vi "PID control - Circle cjehf.vi"() -> ()   [LabVIEW 2017]
uses:
  <vilib>/Simulation/Scripting/Companion Diagram/SimConfigNode/SimParams.ctl
  <vilib>/Simulation/Scripting/Companion Diagram/SimConfigNode/_simSolvers.ctl
  <vilib>/Simulation/Implementation/Shared/SIMSCR Execution Mode.ctl
  <vilib>/Simulation/Param Hierarchy/Typedefs/SIMPH Param Control Actions.ctl
  <vilib>/Simulation/Implementation/Shared/NILVSim_ParamChanged.vi
  <vilib>/Simulation/Implementation/Shared/NILVSIM_BeginStep.vi
  <vilib>/Simulation/Implementation/Shared/NILVSim_Manager.vi
  <vilib>/Utility/error.llb/Clear Errors.vi
  <vilib>/Simulation/Implementation/Shared/NILVSim_FinalizeModel.vi
  <vilib>/DAQmx/read.llb/DAQmx Read (Counter DBL 1Chan 1Samp).vi
  <vilib>/DAQmx/read.llb/DAQmx Read (Digital Bool 1Line 1Point).vi
  917b7e52-755f-4d44-bea8-9e7c9beac24e.vi
  a58f9967-76f1-4ebc-ad3d-26e75a3ca160.vi
  <vilib>/DAQmx/write.llb/DAQmx Write (Analog DBL 1Chan 1Samp).vi
  <vilib>/DAQmx/create/channels.llb/DAQmx Create Channel (AO-Voltage-Basic).vi
  <vilib>/DAQmx/create/channels.llb/DAQmx Create Channel (DI-Digital Input).vi
  <vilib>/DAQmx/create/channels.llb/DAQmx Create Channel (CI-Count Edges).vi
  <vilib>/Simulation/Implementation/Shared/SIM Unbundle Sim Info.vi
  <vilib>/Simulation/Implementation/Shared/NILVSim_Initialize.vi
  <vilib>/Simulation/Utility/Implementation/NILVSim Get Time and IsAcceptedStep.vi
  <vilib>/Simulation/Implementation/Shared/SIMSH Read Queue.vi
  <vilib>/Simulation/Implementation/Shared/NILVSim_GetModelError.vi
  <vilib>/Simulation/Implementation/Shared/SIM Bundle Sim Info.vi
  <vilib>/DAQmx/miscellaneous.llb/DAQmx Fill In Error Info.vi
  <vilib>/Simulation/Implementation/XNodeFramework/SimXNode/SimX.xnode
  <vilib>/Simulation/Model Libraries/PID/SIM PID (Parallel).vi
  <vilib>/Simulation/Model Libraries/PID/SIM PID.vi
  <vilib>/Simulation/Scripting/Companion Diagram/SimConfigNode/SimDog.xnode
  <vilib>/Simulation/Model Libraries/PID/SIM PID (Academic).vi
  <vilib>/Simulation/Implementation/Shared/NI_SIM_Implementation.lvlib
panel:
  out "index":dbl
  out "x check":dbl
  out "stop":bool
  out "y final check":dbl
  out "y check":dbl
  out "array x Length":dbl
  out "X array":dbl[](array[numeric])
  out "array Y length":dbl
  out "Y array":dbl[](array[numeric])
  out "Numeric y":dbl
  out "Numeric x":dbl
  out "Numeric 2":dbl
  in  "Radius":dbl
  out "led check":bool
  in  "check instruc":bool
  out "down 2":bool
  out "down":bool
  out "right":bool
  out "x entered":dbl
  out "y enetred":dbl
  out "greater -1 x":bool
  out "less 1 x":bool
  out "direction selected":dbl
  out "circle reset":bool
  in  "part circle":T1(ring)=enum."a"
  out "at 2f":bool
  out "Step 2J":bool
  out "Step 2H":bool
  out "Shape drawing steps":enum16{"corner", "1st switch", "reverse"}(ring)
  out "Step 2D":bool
  out "Step 2C":bool
  out "c":bool
  in  "height":dbl
  in  "length":dbl
  in  "part":T2(ring)=enum."a"
  out "Step 2A":bool
  out "Step 2B":bool
  in  "Has encoders been reset?":enum16{"don't reset", "reset"}(ring)
  out "x distance currently being travelled":dbl
  out "y distance currently being travelled":dbl
  out "error calced":dbl
  out "p1 dis 2":dbl
  out "p1 dis":dbl
  out "error y":dbl
  out "calc distance y":dbl
  out "calc distanc x":dbl
  out "error x":dbl
  out "reached y":bool
  out "reached x":bool
  out "Numeric":dbl
  in  "Draw rectangle":bool
  in  "Draw circle":bool
  out "In drawing mode":bool
  in  "Right-Down":bool
  in  "Left-Up":bool
  in  "Left-Down":bool
  in  "Right-Up":bool
  in  "right":bool
  in  "left":bool
  in  "motor 2":dbl(slide)=1.5 scale=-10.0..10.0
  in  "down":bool
  in  "up":bool
  in  "Y Length":dbl=30.0
  in  "X Length":dbl=30.0
  in  "Motor 2 encoder":tag="Dev1/ctr1"
  out "Pulses M2":dbl format="%.2f"
  in  "Motor 1 encoder":tag="Dev1/ctr0"
  out "Pulses M1":dbl format="%.2f"
  out "Right":bool
  out "Bottom":bool
  out "Left":bool
  out "Top":bool
  in  "Switch 4/Line 3":tag="Dev1/port0/line3"
  in  "Switch 3/Line 2":tag="Dev1/port0/line2"
  in  "Switch 2/Line 1":tag="Dev1/port0/line1"
  in  "Switch 1/Line 0":tag="Dev1/port0/line0"
  in  "Motor stop":bool
  in  "Motor 1":tag="Dev1/ao0"
  in  "max Voltage":dbl=10.0
  in  "Min Voltage":dbl=-10.0
  in  "Motor 2":tag="Dev1/ao1"
  in  "motor 1":dbl(slide)=1.5 scale=-10.0..10.0
  in  "stop":bool
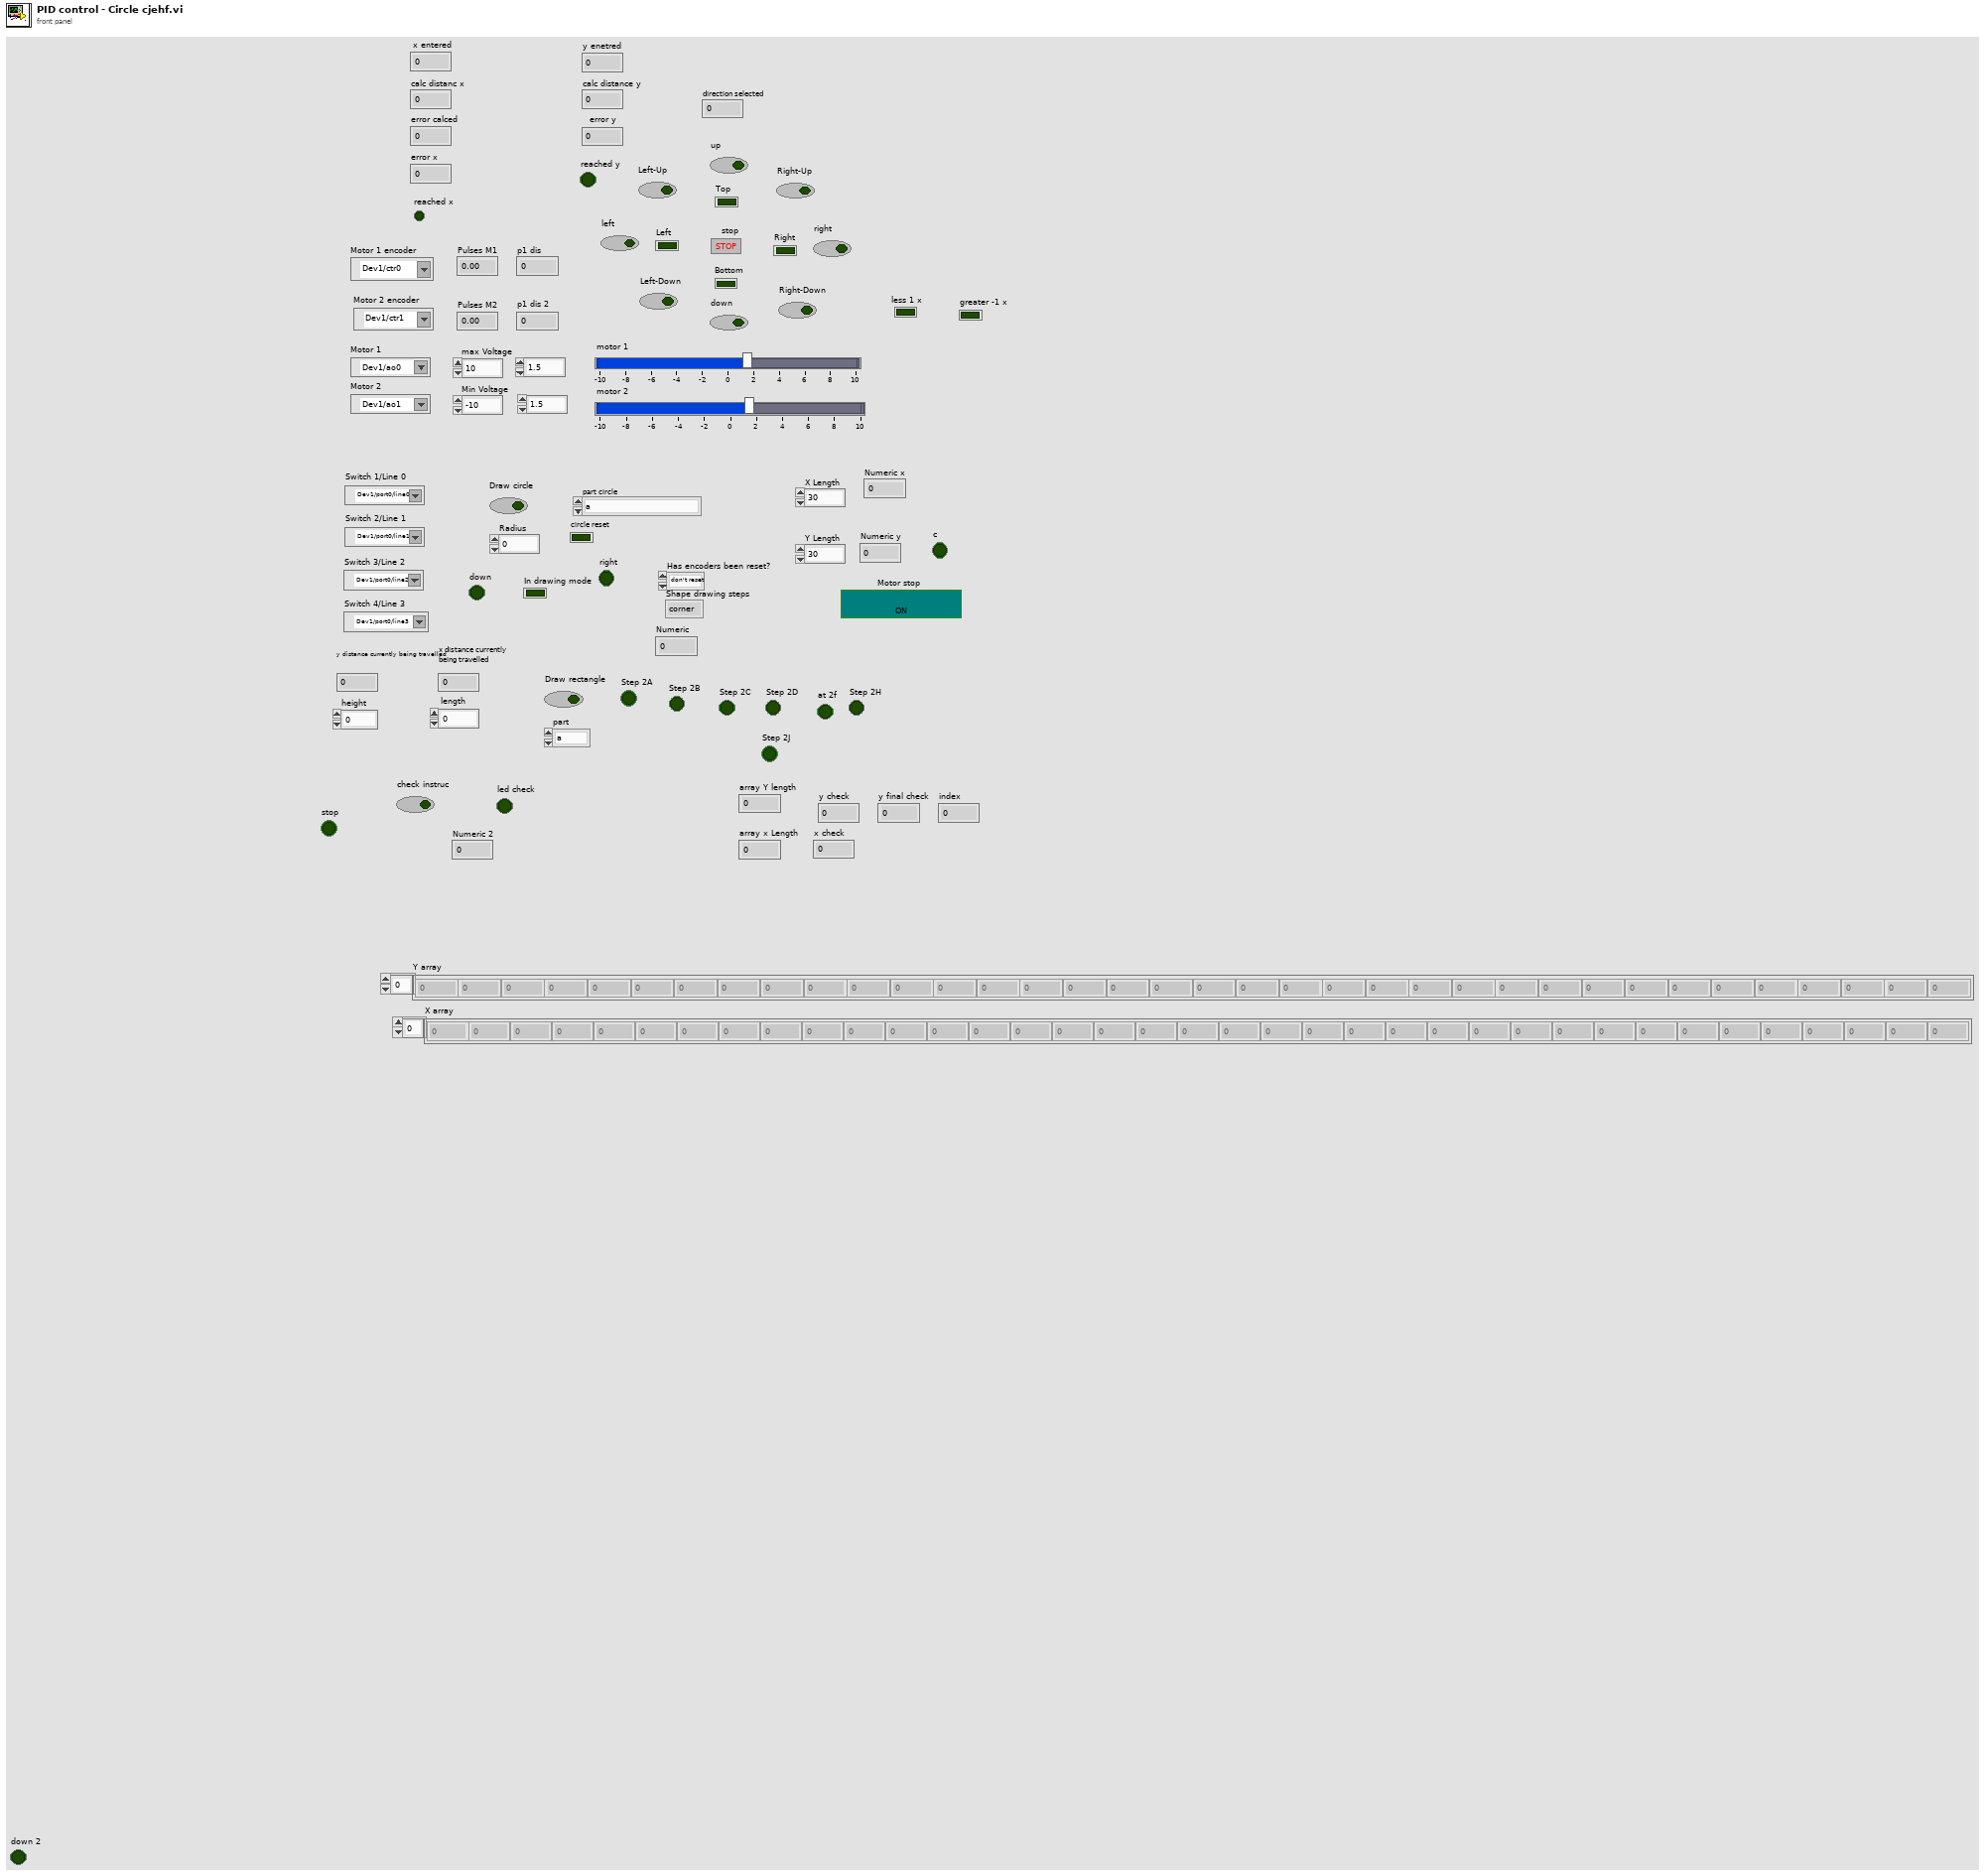
[diagram p1: front panel]
types:
  T1 = enum16{"nothing", "circle", "reset_before_circle", "radius_travel", "going right", "going down", "a"}
  T2 = enum16{"nothing", "j", "i", "h", "g", "f", "e", "d", "c", "b", "a"}
  T3 = enum16{"Simulate to Completion", "Single Time-Step Simulation (Fixed Step Only)"}
  T4 = typedef "SIMSCR Execution Mode.ctl" = enum16{"Simulate to Completion", "Single Time-Step Simulation (Fixed Step Only)"}
  T5 = typedef "SIMPH Param Control Actions.ctl" = enum16{"get params", "set params"}
  T6 = cluster{"SIMSH Sim Time":dbl, "SIM PID Derivative Gain.vi":cluster{"output":dbl}, "SIM PID Derivative Gain.vi - SIMSH":cluster{"SIMSH Sim Time":dbl, "t 3":dbl, "Select 2":cluster{"s? t:f":dbl}, "Equal?":cluster{"x = y?":bool}, "Or":cluster{"x .or. y?":bool}, "Equal To 0?":cluster{"x = 0?":bool}}, "High Frequency [s] (Tf)":dbl, "Gain":cluster{"output":dbl}, "Summation":cluster{"Result":dbl}, "Integral Gain - series.vi":cluster{"output":dbl}, "Integral Gain - series.vi - SIMSH":cluster{"SIMSH Sim Time":dbl, "Select 2":cluster{"s? t:f":dbl}, "integral in gain?":bool, "Integrator":cluster{"output y(t)":dbl}, "Gain 2":cluster{"output":dbl}, "Select":cluster{"s? t:f":dbl}, "Equal To 0?":cluster{"x = 0?":bool}, "Reciprocal":cluster{"1/x":dbl}}}
  T7 = typedef "SimParams.ctl" = cluster{"Initial Time (s)":dbl, "Final Time (s)":dbl, "Step Size (s)":dbl, "ODE Solver":T8, "Minimum Step Size (s)":dbl, "Maximum Step Size (s)":dbl, "Relative Tolerance":dbl, "Absolute Tolerance":dbl, "Software Timing":bool, "Initial Step Size (s)":dbl, "Automatic Fixed Step Size?":bool, "Automatic Discrete Step Size?":bool, "Discrete Step Size (s)":dbl, "Calculate using Time Step":bool, "Solver Wired?":bool, "Prev.Frm.Expected End":u64, "Prev.Frm.Actual End":u64, "Prev.Frm.Finished Late?":bool, "Prev.Iter.Expected End":u64, "Prev.Iter.Actual End":u64, "Prev.Iter.Finished Late?":bool, "Expected Iteration Start":u64, "Actual Iteration Start":u64, "Expected Frame Start":u64, "Actual Frame Start":u64, "Source Name":string, "Name":string, "Period":i64, "Deadline":i64, "Offset":i64, "Start":i64, "Priority":i32, "Timeout":i32, "Processor":i32, "Mode":enum32{"No Change", "Process missed periods, maintain original phase", "Discard missed periods, maintain original phase", "Process missed periods, ignore original phase", "Discard missed periods, ignore original phase"}, "Wakeup reason":enum32{"Normal", "Aborted", "Asynchronous wakeup", "Timing source error", "Timed loop error", "Timeout"}, "Error":errorcluster, "Source Type":string, "Secondary Source Type":string, "Global End Time":u64, "Global Start Time":u64, "Full Solver Reset":bool, "Execution Mode":T4, "Nan/Inf Check":bool, "Custom Solver Library":string, "Solver Is Variable":bool, "custom solver name":string, "Signal Collection Decimation":u32}
  T8 = typedef "_simSolvers.ctl" = enum16{"Runge-Kutta 1 (Euler)", "Runge-Kutta 2", "Runge-Kutta 3", "Runge-Kutta 4", "Runge-Kutta 23 (variable)", "Runge-Kutta 45 (variable)", "BDF (variable)", "Adams-Moulton (variable)", "Rosenbrock (variable)", "Discrete States Only", "SDIRK 4 (variable)", "Radau 5 (variable)", "Radau 9 (variable)", "Radau 13 (variable)", "Radau [Variable Order] (variable)", "Gear's Method (variable)", "Linearizer", "State Query", "Trim Eval", "Custom Solver"}
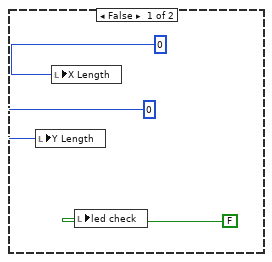
[diagram p2: hidden frame]
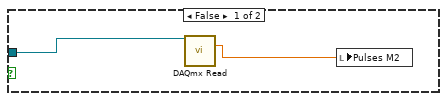
[diagram p3: hidden frame]
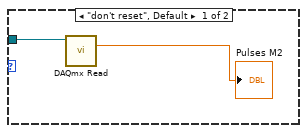
[diagram p4: hidden frame]
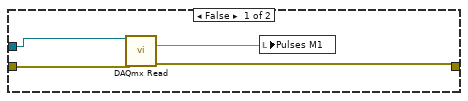
[diagram p5: hidden frame]
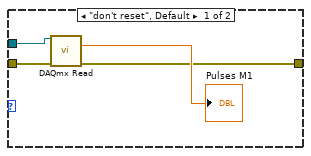
[diagram p6: hidden frame]
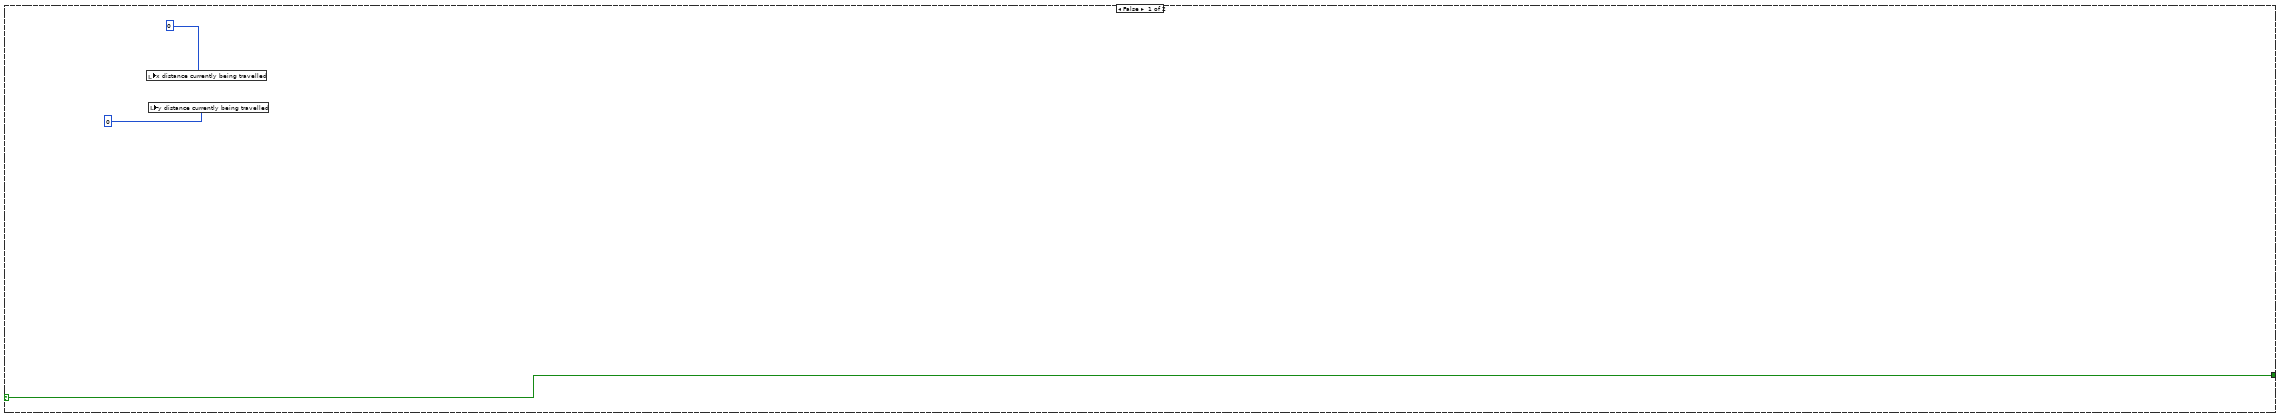
[diagram p7: hidden frame]
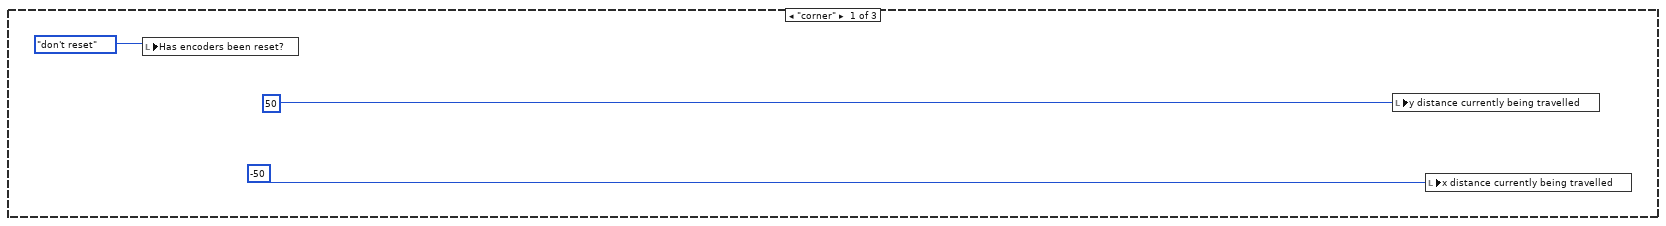
[diagram p8: hidden frame]
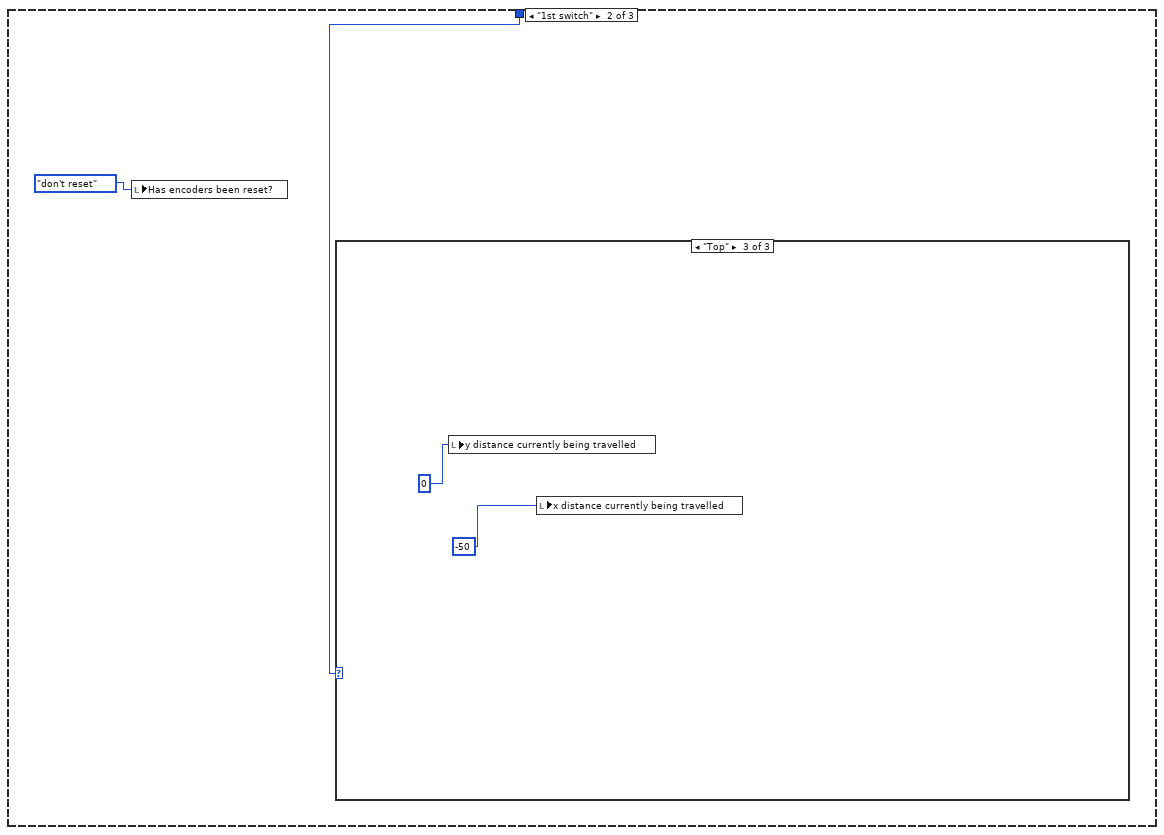
[diagram p9: hidden frame]
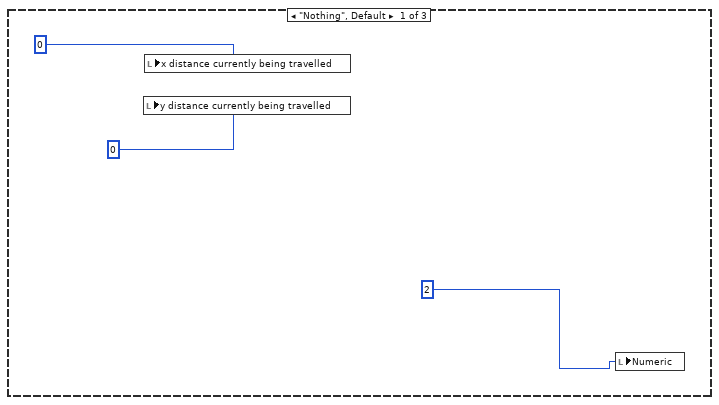
[diagram p10: hidden frame]
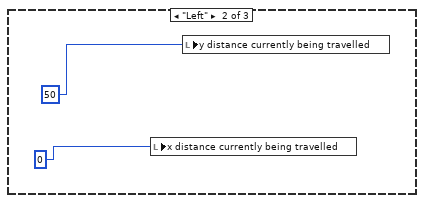
[diagram p11: hidden frame]
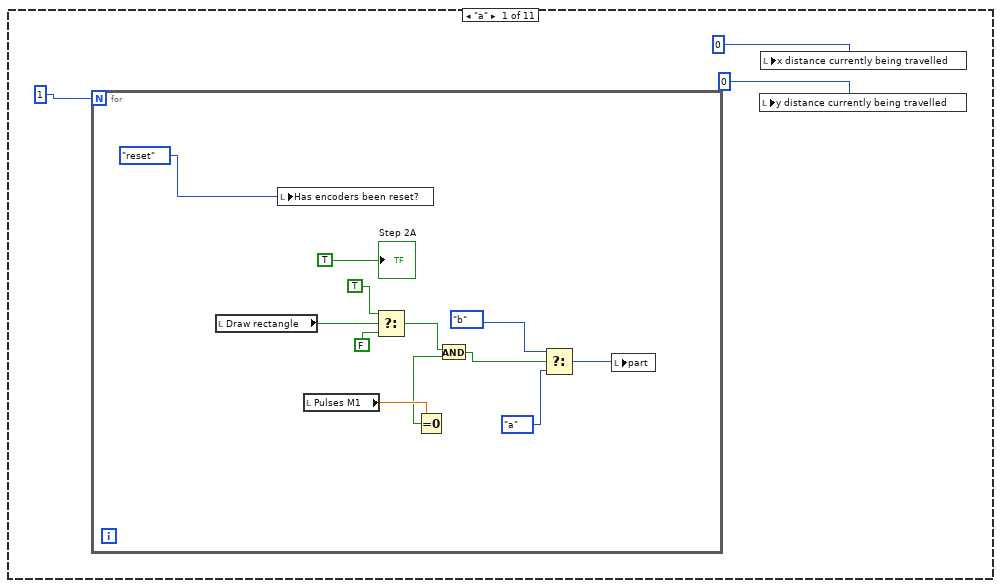
[diagram p12: hidden frame]
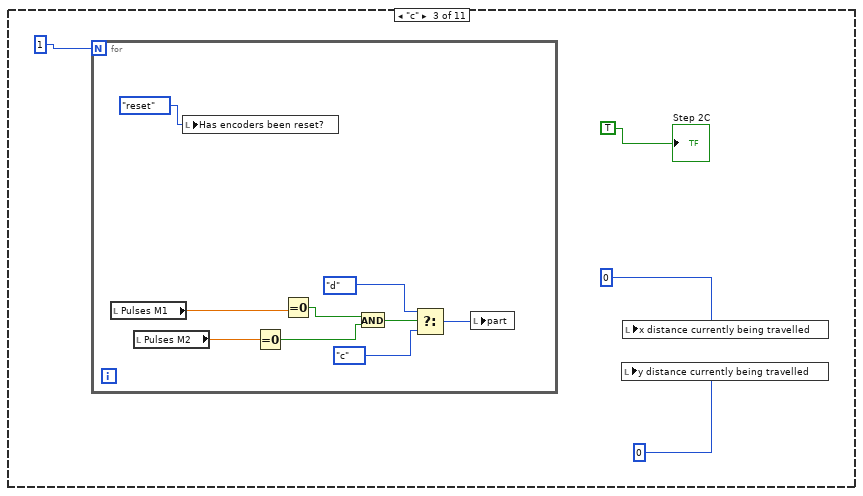
[diagram p13: hidden frame]
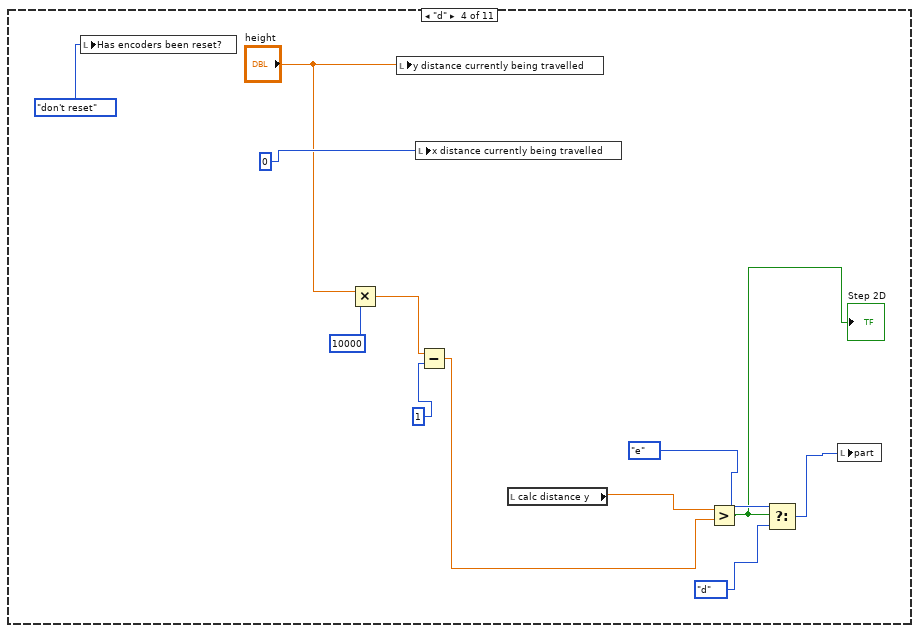
[diagram p14: hidden frame]
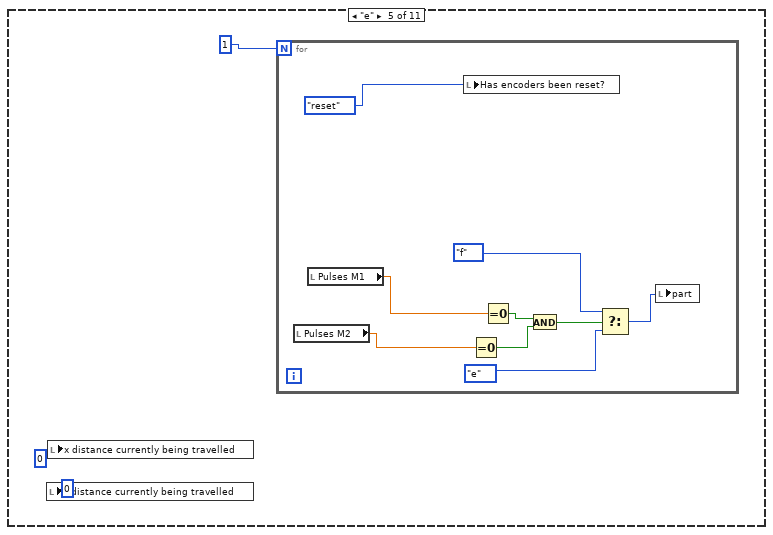
[diagram p15: hidden frame]
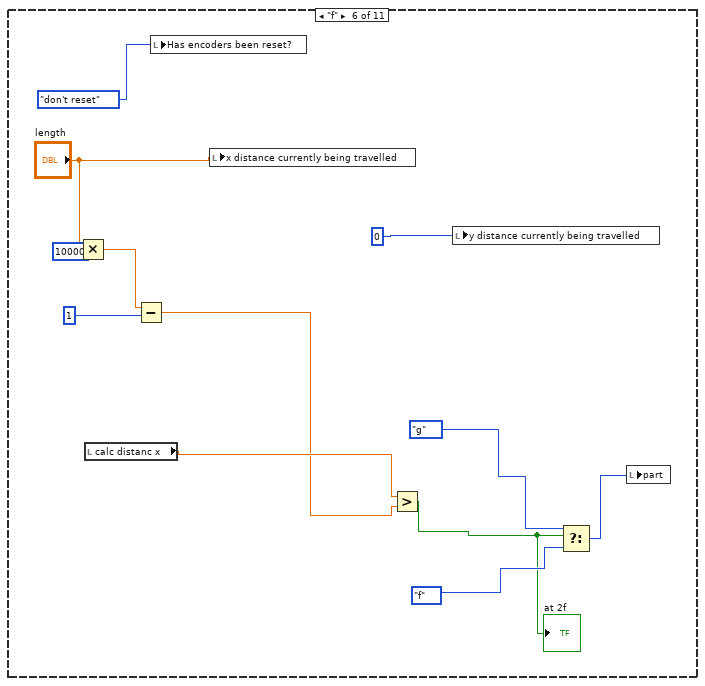
[diagram p16: hidden frame]
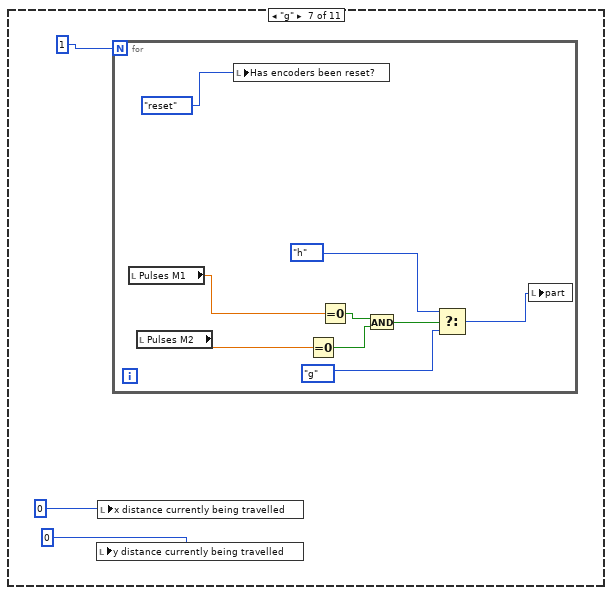
[diagram p17: hidden frame]
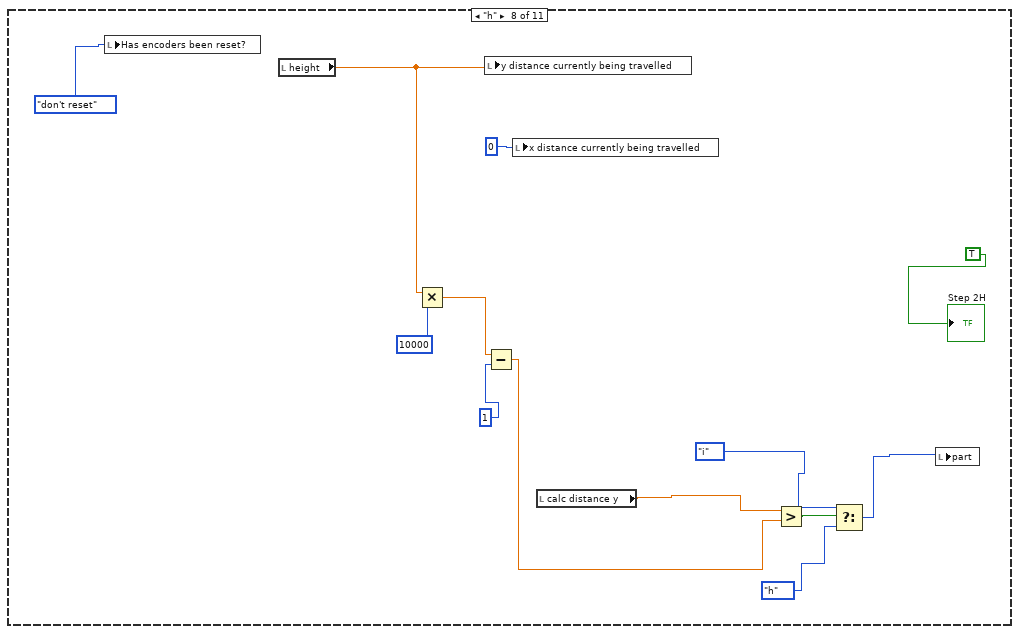
[diagram p18: hidden frame]
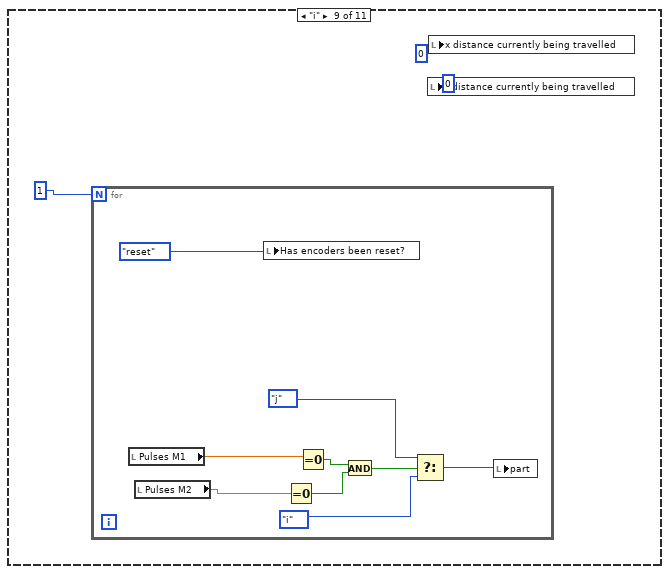
[diagram p19: hidden frame]
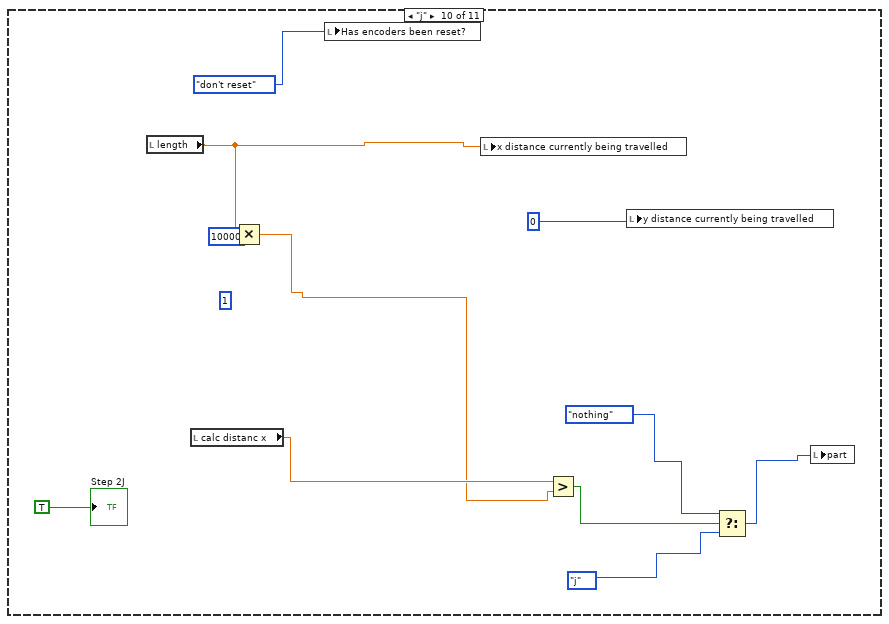
[diagram p20: hidden frame]
diagram:
  n1 = call-poly <vilib>:"DAQmx Create Virtual Channel.vi"("lines"="Switch 1/Line 0") -> ("task out"=w36:refnum<k21>, "error out"=w32:errorcluster)  [unwired: 13 in]
  n2 = call-poly <vilib>:"DAQmx Create Virtual Channel.vi"("lines"="Switch 2/Line 1") -> ("task out"=w35:refnum<k21>, "error out"=w31:errorcluster)  [unwired: 13 in]
  n3 = call-poly <vilib>:"DAQmx Create Virtual Channel.vi"("lines"="Switch 3/Line 2") -> ("task out"=w34:refnum<k21>, "error out"=w30:errorcluster)  [unwired: 13 in]
  n4 = call-poly <vilib>:"DAQmx Create Virtual Channel.vi"("lines"="Switch 4/Line 3") -> ("task out"=w33:refnum<k21>, "error out"=w29:errorcluster)  [unwired: 13 in]
  n5 = call <vilib>:"DAQmx Start Task.vi"("task/channels in"=w36, "error in"=w32) -> ("task out"=w28:refnum<k21>, "error out"=w26:errorcluster)  [unwired: 12 in]
  n6 = call <vilib>:"DAQmx Start Task.vi"("task/channels in"=w35, "error in"=w31) -> ("task out"=w24:refnum<k21>, "error out"=w21:errorcluster)  [unwired: 12 in]
  n7 = call <vilib>:"DAQmx Start Task.vi"("task/channels in"=w34, "error in"=w30) -> ("task out"=w23:refnum<k21>, "error out"=w20:errorcluster)  [unwired: 12 in]
  n8 = call <vilib>:"DAQmx Start Task.vi"("task/channels in"=w33, "error in"=w29) -> ("task out"=w22:refnum<k21>, "error out"=w19:errorcluster)  [unwired: 12 in]
  n9 = call-poly <vilib>:"DAQmx Create Virtual Channel.vi"("maximum value"="max Voltage", "minimum value"="Min Voltage", "physical channels"="Motor 1") -> ("task out"=w46:refnum<k21>, "error out"=w42:errorcluster)  [unwired: 11 in]
  n10 = call-poly <vilib>:"DAQmx Create Virtual Channel.vi"("counter"="Motor 2 encoder") -> ("task out"=w6:refnum<k21>)  [unwired: 13 in, 1 out]
  n11 = call-poly <vilib>:"DAQmx Create Virtual Channel.vi"("maximum value"="max Voltage", "minimum value"="Min Voltage", "physical channels"="Motor 2") -> ("task out"=w49:refnum<k21>, "error out"=w41:errorcluster)  [unwired: 11 in]
  n12 = call-poly <vilib>:"DAQmx Create Virtual Channel.vi"("counter"="Motor 1 encoder") -> ("task out"=w7:refnum<k21>, "error out"=w2:errorcluster)  [unwired: 13 in]
  n13 = call <vilib>:"DAQmx Start Task.vi"("task/channels in"=w6) -> ("task out"=w1:refnum<k21>)  [unwired: 13 in, 1 out]
  n14 = call <vilib>:"DAQmx Start Task.vi"("task/channels in"=w7) -> ("task out"=w3:refnum<k21>)  [unwired: 13 in, 1 out]
  n15 = while {
    tunnel: w49 -> [w236]
    tunnel: [w233] -> w48
    tunnel: w46 -> [w230]
    tunnel: [w229] -> w45
    tunnel: w42 -> [w227]
    tunnel: w41 -> [w226]
    tunnel: w28 -> [w220]
    tunnel: [w219] -> w27
    tunnel: w26 -> [w218]
    tunnel: [w217] -> w25
    tunnel: w24 -> [w216]
    tunnel: w23 -> [w215]
    tunnel: w22 -> [w214]
    tunnel: w21 -> [w213]
    tunnel: w20 -> [w212]
    tunnel: w19 -> [w211]
    tunnel: [w210] -> w18
    tunnel: [w209] -> w17
    tunnel: [w208] -> w16
    tunnel: [w207] -> w15
    tunnel: [w206] -> w14
    tunnel: [w205] -> w13
    tunnel: [w139] -> w10
    tunnel: w3 -> [w141]
    tunnel: w2 -> [w140]
    tunnel: w1 -> [w137]
    stop <- "stop" stop-if-true
    (unwired) TRUE
    n16 = Or(x="Draw circle", y="Draw rectangle") -> (x .or. y?=w149:bool)
    n17 = case shown="True" "check instruc" {
      frame False {
        n18 = local write "Y Length"(0) -> ()
        n19 = local write "X Length"(0) -> ()
        n20 = local write "led check"(FALSE) -> ()
      }
      frame True {
        n21 = flat-sequence {
          frame #0 {
            n22 = while {
              stop <- w246 stop-if-true
              n23 = for {
                N: 50 -> [_]
                shift-right: [w252] -> w245
                shift-left: _ -> [_]
                tunnel: [w252] -> w240 mode=indexing
                shift-right: [w251] -> w243
                shift-left: _ -> [_]
                tunnel: [w251] -> w241 mode=indexing
                i -> [w254]
                n24 = Multiply(x=2, y=3.141592653589793) -> (x*y=w258:dbl)
                n25 = Increment(x=w254) -> (x+1=w256:i32)
                n26 = Divide(x=w258, y=50) -> (x/y=w260:dbl)
                n27 = Multiply(x=w260, y=w256) -> (x*y=w257:dbl)
                n28 = local write "led check"(TRUE) -> ()
                n29 = local write "Has encoders been reset?"(enum16{"don't reset", "reset"}."don't reset") -> ()
                n30 = Cosine(x=w257) -> (cos(x)=w263:dbl)
                n31 = Sine(x=w257) -> (sin(x)=w264:dbl)
                n32 = Multiply(x=w264, y="Radius") -> (x*y=w252:dbl)
                n33 = Multiply(x=w263, y="Radius") -> (x*y=w251:dbl)
                "Numeric 2" <- w254
              }
              "Numeric y" <- w245
              "Y array" <- w240
              "Numeric x" <- w243
              "X array" <- w241
              n34 = local read "Numeric 2"() -> (w248:dbl)
              n35 = Equal?(x=w248, y=49) -> (x = y?=w246:bool)
              n36 = Array Size(array=w240) -> (size(s)=→"array Y length":i32)
              n37 = Array Size(array=w241) -> (size(s)=→"array x Length":i32)
            }
          }
          frame #1 {
            n38 = flat-sequence {
              tunnel: [w269] -> w268
              tunnel: w265 -> [w269]
              tunnel: w268 -> [w276]
              tunnel: [w278] -> w267
              tunnel: [w277] -> w266
              frame #0 {
                n39 = local read "Y array"() -> (w273:dbl[])
                n40 = local read "X array"() -> (w271:dbl[])
                n41 = Index Array(array=w271, index=w269) -> (element=w270:dbl)
                "x check" <- w270
                n42 = Index Array(array=w273, index=w269) -> (element=w272:dbl)
                "y check" <- w272
                n43 = local write "X Length"(w270) -> ()
                n44 = local write "Y Length"(w272) -> ()
              }
              frame #1 {
                n45 = local read "calc distance y"() -> (w287:dbl)
                n46 = local read "calc distanc x"() -> (w283:dbl)
                n47 = local read "index"() -> (w275:dbl)
                n48 = Greater?(x=w287, y=1000) -> (0:w280:bool)
                n49 = Greater?(x=w283, y=1000) -> (0:w281:bool)
                n50 = And(x=w280, y=w281) -> (x .and. y?=w279:bool)
                n51 = Increment(x=w275) -> (x+1=w274:dbl)
                n52 = Select(t=w274, s=w279, f=w276) -> (s? t:f=w277:dbl)
                "y final check" <- w277
                n53 = Equal?(x=w277, y=50) -> (x = y?=w278:bool)
                "led check" <- TRUE
              }
            }
            n54 = feedback-in #1(w266) -> ()
            n55 = feedback #1() -> (w265:dbl)  [unwired: 1 in]
            "index" <- w265
            "stop" <- w267
          }
        }
      }
    }
    n56 = local read "error y"() -> (w108:dbl)
    n57 = local read "error y"() -> (w107:dbl)
    n58 = local read "error x"() -> (w109:dbl)
    n59 = local read "error y"() -> (w123:dbl)
    n60 = local read "error y"() -> (w120:dbl)
    n61 = local read "error x"() -> (w116:dbl)
    n62 = local read "error x"() -> (w115:dbl)
    n63 = local read "error y"() -> (w124:dbl)
    n64 = local read "error x"() -> (w125:dbl)
    n65 = Less Than 0?(x=w108) -> (x < 0?=w106:bool)
    n66 = Less Than 0?(x=w109) -> (x < 0?=w105:bool)
    n67 = Greater Than 0?(x=w107) -> (x > 0?=w104:bool)
    n68 = Less Than 0?(x=w120) -> (x < 0?=w118:bool)
    n69 = Equal To 0?(x=w125) -> (x = 0?=w119:bool)
    n70 = Greater Than 0?(x=w123) -> (x > 0?=w122:bool)
    n71 = local read "error y"() -> (w101:dbl)
    n72 = local read "error x"() -> (w100:dbl)
    n73 = Greater Than 0?(x=w116) -> (x > 0?=w114:bool)
    n74 = Equal To 0?(x=w124) -> (x = 0?=w113:bool)
    n75 = Less Than 0?(x=w115) -> (x < 0?=w112:bool)
    n76 = And(x=w106, y=w105) -> (x .and. y?=w102:bool)
    n77 = And(x=w105, y=w104) -> (x .and. y?=w103:bool)
    n78 = And(x=w122, y=w119) -> (x .and. y?=w121:bool)
    n79 = And(x=w119, y=w118) -> (x .and. y?=w117:bool)
    n80 = local read "error y"() -> (w96:dbl)
    n81 = And(x=w114, y=w113) -> (x .and. y?=w111:bool)
    n82 = And(x=w113, y=w112) -> (x .and. y?=w110:bool)
    n83 = Greater Than 0?(x=w101) -> (x > 0?=w99:bool)
    n84 = Greater Than 0?(x=w100) -> (x > 0?=w97:bool)
    n85 = Less Than 0?(x=w96) -> (x < 0?=w95:bool)
    n86 = And(x=w99, y=w97) -> (x .and. y?=w98:bool)
    n87 = And(x=w97, y=w95) -> (x .and. y?=w94:bool)
    n88 = Select(t=1, s=w121, f=0) -> (s? t:f=w189:i32)
    n89 = Select(t=10, s=w110, f=0) -> (s? t:f=w187:i32)
    n90 = Select(t=2, s=w117, f=0) -> (s? t:f=w188:i32)
    n91 = Select(t=100, s=w98, f=0) -> (s? t:f=w185:i32)
    n92 = Select(t=200, s=w102, f=0) -> (s? t:f=w184:i32)
    n93 = Select(t=20, s=w111, f=0) -> (s? t:f=w186:i32)
    n94 = Select(t=1000, s=w103, f=0) -> (s? t:f=w183:i32)
    n95 = Select(t=2000, s=w94, f=0) -> (s? t:f=w169:i32)
    n96 = Add(x=w189, y=w188) -> (x+y=w182:i32)
    n97 = Add(x=w187, y=w186) -> (x+y=w181:i32)
    n98 = Add(x=w185, y=w184) -> (x+y=w180:i32)
    n99 = Add(x=w183, y=w169) -> (x+y=w168:i32)
    n100 = local read "y check"() -> (w51:dbl)
    n101 = Add(x=w182, y=w181) -> (x+y=w179:i32)
    n102 = Add(x=w180, y=w168) -> (x+y=w167:i32)
    n103 = call-poly <vilib>:"DAQmx Read.vi"("task/channels in"=w220, "error in"=w218) -> ("task out"=w219:refnum<k21>, "data"=w151:bool, "error out"=w217:errorcluster)  [unwired: 11 in]
    "Top" <- w151
    n104 = call-poly <vilib>:"DAQmx Read.vi"("task/channels in"=w216, "error in"=w213) -> ("task out"=w210:refnum<k21>, "data"=w160:bool, "error out"=w207:errorcluster)  [unwired: 11 in]
    "Bottom" <- w160
    n105 = call-poly <vilib>:"DAQmx Read.vi"("task/channels in"=w215, "error in"=w212) -> ("task out"=w209:refnum<k21>, "data"=w159:bool, "error out"=w206:errorcluster)  [unwired: 11 in]
    "Right" <- w159
    n106 = call-poly <vilib>:"DAQmx Read.vi"("task/channels in"=w214, "error in"=w211) -> ("task out"=w208:refnum<k21>, "data"=w158:bool, "error out"=w205:errorcluster)  [unwired: 11 in]
    "Left" <- w158
    n107 = Add(x=w179, y=w167) -> (x+y=w93:i32)
    "direction selected" <- w93
    n108 = local read "check instruc"() -> (w52:bool)
    n109 = Select(t=w51, s=w52, f="Y Length") -> (s? t:f=w53:dbl)
    n110 = Multiply(x=w53, y=10) -> (x*y=w55:dbl)
    "y enetred" <- w55
    n111 = local read "Pulses M1"() -> (w138:dbl)
    n112 = local read "Pulses M2"() -> (w142:dbl)
    n113 = Divide(x=w138, y=52.56) -> (x/y=→"p1 dis":dbl)
    n114 = feedback #2() -> (w67:dbl)  [unwired: 1 in]
    "calc distance y" <- w67
    n115 = formula code="if (Ylength==0)\nYerror=0;\n else  \nif(Ylength<0)\nYerror= Ylength+calculating_y_dis;\nelse\nYerror= Ylength-calculating_y_dis;\n\nif (calculating_y_dis>1000)\nstay=0;\nif (stay==0 )\nYerror=0;"("Ylength"=w55, "calculating_y_dis"=w67, "stay"=1) -> ("Yerror"=w127:dbl)
    n116 = Divide(x=w142, y=52.56) -> (x/y=→"p1 dis 2":dbl)
    n117 = formula code="X=((PulseM1/52.56)+(PulseM2/52.56))/2.0;\nY=((PulseM1/52.56)+(PulseM2/52.56))/2.0;"("PulseM1"=w138, "PulseM2"=w142) -> ("X"=w72:dbl, "Y"=w76:dbl)
    n118 = local read "check instruc"() -> (w58:bool)
    n119 = Multiply(x=1000, y=w76) -> (x*y=w79:dbl)
    n120 = xnode "PID"("Error"=w127) -> ("Output"=w78:dbl)  [unwired: 2 in, 11 out]
    n121 = local read "x check"() -> (w59:dbl)
    n122 = Select(t=w59, s=w58, f="X Length") -> (s? t:f=w56:dbl)
    n123 = Multiply(x=w56, y=10) -> (x*y=w63:dbl)
    "x entered" <- w63
    n124 = Multiply(x=1000, y=w72) -> (x*y=w73:dbl)
    n125 = Greater?(x=1, y=w78) -> (0:w91:bool)
    n126 = Less?(x=-1, y=w78) -> (x < y?=w89:bool)
    n127 = case shown="2000" w93 {
      tunnel: "motor 1" -> [w1022 w1025 w1028 w1035 w1039 w1043 w1049 w1055 w1061 w1066 w1073]
      tunnel: "motor 2" -> [w1019 w1027 w1030 w1033 w1038 w1041 w1047 w1053 w1059 w1067 w1072]
      tunnel: [w1018 w1027 w1029 w1032 w1038 w1040 w1046 w1052 w1058 w1064 w1071] -> w61
      tunnel: [w1021 w1024 w1028 w1034 w1039 w1042 w1048 w1054 w1060 w1065 w1070] -> w62
      frame 0, Default {
        n128 = Multiply(x=0, y=w1022) -> (x*y=w1021:dbl)
        n129 = Multiply(x=0, y=w1019) -> (x*y=w1018:dbl)
      }
      frame 1 {
        n130 = Multiply(x=-1, y=w1025) -> (x*y=w1024:dbl)
      }
      frame 2 {
        n131 = Multiply(x=-1.003, y=w1030) -> (x*y=w1029:dbl)
      }
      frame 10 {
        n132 = Multiply(x=-1, y=w1035) -> (x*y=w1034:dbl)
        n133 = Multiply(x=-1.1, y=w1033) -> (x*y=w1032:dbl)
      }
      frame 20 {
      }
      frame 100 {
        n134 = Multiply(x=0, y=w1043) -> (x*y=w1042:dbl)
        n135 = Multiply(x=1, y=w1041) -> (x*y=w1040:dbl)
      }
      frame 200 {
        n136 = Multiply(x=0, y=w1049) -> (x*y=w1048:dbl)
        n137 = Multiply(x=-1, y=w1047) -> (x*y=w1046:dbl)
      }
      frame 1000 {
        n138 = Multiply(x=-1, y=w1055) -> (x*y=w1054:dbl)
        n139 = Multiply(x=0, y=w1053) -> (x*y=w1052:dbl)
      }
      frame 2000 {
        n140 = Multiply(x=1, y=w1061) -> (x*y=w1060:dbl)
        n141 = Multiply(x=0, y=w1059) -> (x*y=w1058:dbl)
      }
      frame 4000 {
        n142 = Multiply(x=-1, y=w1066) -> (x*y=w1065:dbl)
        n143 = Multiply(x=0, y=w1067) -> (x*y=w1064:dbl)
      }
      frame 8000 {
        n144 = Multiply(x=-1, y=w1073) -> (x*y=w1070:dbl)
        n145 = Multiply(x=0, y=w1072) -> (x*y=w1071:dbl)
      }
    }
    n146 = And(x=w91, y=w89) -> (x .and. y?=w77:bool)
    "reached y" <- w77
    n147 = Select(t=w79, s=w77, f=w76) -> (s? t:f=w75:dbl)
    n148 = feedback-in #2(w75) -> ()
    n149 = Multiply(x=0, y=w78) -> (x*y=w87:dbl)
    n150 = Select(t=w87, s=w77, f=w78) -> (s? t:f=→"error y":dbl)
    n151 = local read "Numeric"() -> (w131:dbl)
    n152 = Or(x=w160, y=w159) -> (x .or. y?=w203:bool)
    n153 = local read "Draw circle"() -> (w135:bool)
    n154 = local read "Draw rectangle"() -> (w134:bool)
    n155 = And(x=w158, y=w151) -> (x .and. y?=w132:bool)
    n156 = Exclusive Or(1:w151, 2:w158) -> (0:w165:bool)
    n157 = Select(t=1, s=w158, f=0) -> (s? t:f=w150:i32)
    n158 = Select(t=2, s=w151, f=w150) -> (s? t:f=w155:i32)
    n159 = Select(t=1, s=w165, f=w131) -> (s? t:f=w164:dbl)
    n160 = Select(t=2, s=w132, f=w164) -> (s? t:f=w162:dbl)
    n161 = feedback #3() -> (w70:bool)  [unwired: 1 in]
    "reached x" <- w70
    n162 = Select(t=w73, s=w70, f=w72) -> (s? t:f=w66:dbl)
    "calc distanc x" <- w66
    n163 = formula code="if (desired_xlength==0)\nXerror=0;\nelse\nif(desired_xlength>0)\nXerror=desired_xlength-actual_xLength;\nelse\nXerror=desired_xlength+actual_xLength;\n\nif (actual_xLength>1000)\nstay1=0;\nif (stay1==0)\nXerror=0;"("actual_xLength"=w66, "desired_xlength"=w63, "stay1"=1) -> ("Xerror"=w126:dbl)
    "error calced" <- w126
    n164 = xnode "PID 2"("Error"=w126) -> ("Output"=w82:dbl)  [unwired: 2 in, 11 out]
    n165 = Greater?(x=1, y=w82) -> (0:w68:bool)
    "greater -1 x" <- w68
    n166 = Less?(x=-1, y=w82) -> (x < y?=w69:bool)
    "less 1 x" <- w69
    n167 = And(x=w68, y=w69) -> (x .and. y?=w71:bool)
    n168 = Multiply(x=0, y=w82) -> (x*y=w84:dbl)
    n169 = feedback-in #3(w71) -> ()
    n170 = Or(x=w135, y=w134) -> (x .or. y?=w136:bool)
    n171 = Select(t=w84, s=w70, f=w82) -> (s? t:f=→"error x":dbl)
    n172 = call "Number To Enum.vim"("number"=w155, "enum type"=enum16{"Nothing", "Left", "Top"}."Nothing") -> ("number as enum"=w152:enum16{"Nothing", "Left", "Top"})
    n173 = case shown="True" w149 {
      selector: w149 -> [w814 w822]
      tunnel: [w814 w822] -> w166
      tunnel: w152 -> [_ w815]
      frame False {
        n174 = local write "x distance currently being travelled"(0) -> ()
        n175 = local write "y distance currently being travelled"(0) -> ()
      }
      frame True {
        n176 = local read "Numeric"() -> (w820:dbl)
        n177 = local read "Shape drawing steps"() -> (w817:enum16{"corner", "1st switch", "reverse"})
        n178 = Equal?(x=w820, y=2) -> (x = y?=w819:bool)
        n179 = Select(t=enum16{"corner", "1st switch", "reverse"}."reverse", s=w819, f=w817) -> (s? t:f=w816:enum16{"corner", "1st switch", "reverse"})
        n180 = case shown="\"reverse\"" w816 {
          tunnel: w815 -> [_ w826 _]
          frame "corner" {
            n181 = local write "Has encoders been reset?"(enum16{"don't reset", "reset"}."don't reset") -> ()
            n182 = local write "y distance currently being travelled"(50) -> ()
            n183 = local write "x distance currently being travelled"(-50) -> ()
          }
          frame "1st switch" {
            n184 = local write "Has encoders been reset?"(enum16{"don't reset", "reset"}."don't reset") -> ()
            n185 = case shown="\"Top\"" w826 {
              frame "Nothing", Default {
                n186 = local write "y distance currently being travelled"(0) -> ()
                n187 = local write "x distance currently being travelled"(0) -> ()
                n188 = local write "Numeric"(2) -> ()
              }
              frame "Left" {
                n189 = local write "x distance currently being travelled"(0) -> ()
                n190 = local write "y distance currently being travelled"(50) -> ()
              }
              frame "Top" {
                n191 = local write "y distance currently being travelled"(0) -> ()
                n192 = local write "x distance currently being travelled"(-50) -> ()
              }
            }
          }
          frame "reverse" {
            n193 = local read "Draw circle"() -> (w835:bool)
            n194 = case shown="False" w835 {
              tunnel: "part" -> [w838 _]
              frame False {
                n195 = case shown="\"b\"" w838 {
                  frame "a" {
                    n196 = for {
                      N: 1 -> [_]
                      n197 = local read "Draw rectangle"() -> (w842:bool)
                      n198 = local write "Has encoders been reset?"(enum16{"don't reset", "reset"}."reset") -> ()
                      n199 = local read "Pulses M1"() -> (w851:dbl)
                      n200 = Select(t=TRUE, s=w842, f=FALSE) -> (s? t:f=w845:bool)
                      n201 = Equal To 0?(x=w851) -> (x = 0?=w844:bool)
                      n202 = And(x=w845, y=w844) -> (x .and. y?=w843:bool)
                      n203 = Select(t=T2."b", s=w843, f=T2."a") -> (s? t:f=w850:T2)
                      n204 = local write "part"(w850) -> ()
                      "Step 2A" <- TRUE
                    }
                    n205 = local write "y distance currently being travelled"(0) -> ()
                    n206 = local write "x distance currently being travelled"(0) -> ()
                  }
                  frame "b" {
                    n207 = local read "calc distance y"() -> (w854:dbl)
                    n208 = local read "calc distanc x"() -> (w855:dbl)
                    n209 = local write "Has encoders been reset?"(enum16{"don't reset", "reset"}."don't reset") -> ()
                    n210 = Greater?(x=w854, y=9000) -> (0:w860:bool)
                    n211 = Greater?(x=w855, y=29000) -> (0:w859:bool)
                    n212 = And(x=w859, y=w860) -> (x .and. y?=w858:bool)
                    "c" <- w858
                    n213 = Select(t=T2."c", s=w858, f=T2."b") -> (s? t:f=w863:T2)
                    n214 = local write "part"(w863) -> ()
                    "x distance currently being travelled" <- 3
                    "y distance currently being travelled" <- 1
                    "Step 2B" <- TRUE
                  }
                  frame "c" {
                    n215 = for {
                      N: 1 -> [_]
                      n216 = local read "Pulses M1"() -> (w879:dbl)
                      n217 = local read "Pulses M2"() -> (w875:dbl)
                      n218 = local write "Has encoders been reset?"(enum16{"don't reset", "reset"}."reset") -> ()
                      n219 = Equal To 0?(x=w875) -> (x = 0?=w873:bool)
                      n220 = Equal To 0?(x=w879) -> (x = 0?=w874:bool)
                      n221 = And(x=w874, y=w873) -> (x .and. y?=w872:bool)
                      n222 = Select(t=T2."d", s=w872, f=T2."c") -> (s? t:f=w878:T2)
                      n223 = local write "part"(w878) -> ()
                    }
                    n224 = local write "y distance currently being travelled"(0) -> ()
                    n225 = local write "x distance currently being travelled"(0) -> ()
                    "Step 2C" <- TRUE
                  }
                  frame "d" {
                    n226 = local write "Has encoders been reset?"(enum16{"don't reset", "reset"}."don't reset") -> ()
                    n227 = Multiply(x="height", y=10000) -> (x*y=w888:dbl)
                    n228 = local write "y distance currently being travelled"("height") -> ()
                    n229 = local write "x distance currently being travelled"(0) -> ()
                    n230 = Subtract(x=w888, y=1) -> (x-y=w885:dbl)
                    n231 = local read "calc distance y"() -> (w890:dbl)
                    n232 = Greater?(x=w890, y=w885) -> (0:w881:bool)
                    "Step 2D" <- w881
                    n233 = Select(t=T2."e", s=w881, f=T2."d") -> (s? t:f=w891:T2)
                    n234 = local write "part"(w891) -> ()
                  }
                  frame "e" {
                    n235 = local write "y distance currently being travelled"(0) -> ()
                    n236 = local write "x distance currently being travelled"(0) -> ()
                    n237 = for {
                      N: 1 -> [_]
                      n238 = local read "Pulses M2"() -> (w897:dbl)
                      n239 = local read "Pulses M1"() -> (w898:dbl)
                      n240 = local write "Has encoders been reset?"(enum16{"don't reset", "reset"}."reset") -> ()
                      n241 = Equal To 0?(x=w897) -> (x = 0?=w903:bool)
                      n242 = Equal To 0?(x=w898) -> (x = 0?=w904:bool)
                      n243 = And(x=w904, y=w903) -> (x .and. y?=w902:bool)
                      n244 = Select(t=T2."f", s=w902, f=T2."e") -> (s? t:f=w896:T2)
                      n245 = local write "part"(w896) -> ()
                    }
                  }
                  frame "f" {
                    n246 = Multiply(x="length", y=10000) -> (x*y=w911:dbl)
                    n247 = local read "calc distanc x"() -> (w914:dbl)
                    n248 = Subtract(x=w911, y=1) -> (x-y=w908:dbl)
                    n249 = local write "Has encoders been reset?"(enum16{"don't reset", "reset"}."don't reset") -> ()
                    n250 = local write "x distance currently being travelled"("length") -> ()
                    n251 = Greater?(x=w914, y=w908) -> (0:w905:bool)
                    "at 2f" <- w905
                    n252 = local write "y distance currently being travelled"(0) -> ()
                    n253 = Select(t=T2."g", s=w905, f=T2."f") -> (s? t:f=w913:T2)
                    n254 = local write "part"(w913) -> ()
                  }
                  frame "g" {
                    n255 = local write "y distance currently being travelled"(0) -> ()
                    n256 = local write "x distance currently being travelled"(0) -> ()
                    n257 = for {
                      N: 1 -> [_]
                      n258 = local read "Pulses M1"() -> (w921:dbl)
                      n259 = local read "Pulses M2"() -> (w920:dbl)
                      n260 = local write "Has encoders been reset?"(enum16{"don't reset", "reset"}."reset") -> ()
                      n261 = Equal To 0?(x=w920) -> (x = 0?=w927:bool)
                      n262 = Equal To 0?(x=w921) -> (x = 0?=w928:bool)
                      n263 = And(x=w928, y=w927) -> (x .and. y?=w926:bool)
                      n264 = Select(t=T2."h", s=w926, f=T2."g") -> (s? t:f=w923:T2)
                      n265 = local write "part"(w923) -> ()
                    }
                  }
                  frame "h" {
                    n266 = local write "Has encoders been reset?"(enum16{"don't reset", "reset"}."don't reset") -> ()
                    n267 = local read "height"() -> (w932:dbl)
                    n268 = Multiply(x=w932, y=10000) -> (x*y=w940:dbl)
                    n269 = local write "y distance currently being travelled"(w932) -> ()
                    n270 = Subtract(x=w940, y=1) -> (x-y=w937:dbl)
                    n271 = local write "x distance currently being travelled"(0) -> ()
                    n272 = local read "calc distance y"() -> (w930:dbl)
                    n273 = Greater?(x=w930, y=w937) -> (0:w941:bool)
                    n274 = Select(t=T2."i", s=w941, f=T2."h") -> (s? t:f=w933:T2)
                    n275 = local write "part"(w933) -> ()
                    "Step 2H" <- TRUE
                  }
                  frame "i" {
                    n276 = for {
                      N: 1 -> [_]
                      n277 = local read "Pulses M1"() -> (w947:dbl)
                      n278 = local read "Pulses M2"() -> (w946:dbl)
                      n279 = local write "Has encoders been reset?"(enum16{"don't reset", "reset"}."reset") -> ()
                      n280 = Equal To 0?(x=w946) -> (x = 0?=w952:bool)
                      n281 = Equal To 0?(x=w947) -> (x = 0?=w953:bool)
                      n282 = And(x=w953, y=w952) -> (x .and. y?=w951:bool)
                      n283 = Select(t=T2."j", s=w951, f=T2."i") -> (s? t:f=w945:T2)
                      n284 = local write "part"(w945) -> ()
                    }
                    n285 = local write "y distance currently being travelled"(0) -> ()
                    n286 = local write "x distance currently being travelled"(0) -> ()
                  }
                  frame "j" {
                    (unwired) 1
                    n287 = local read "length"() -> (w957:dbl)
                    n288 = local read "calc distanc x"() -> (w959:dbl)
                    n289 = Multiply(x=w957, y=10000) -> (x*y=w954:dbl)
                    n290 = local write "Has encoders been reset?"(enum16{"don't reset", "reset"}."don't reset") -> ()
                    n291 = local write "x distance currently being travelled"(w957) -> ()
                    n292 = Greater?(x=w959, y=w954) -> (0:w962:bool)
                    n293 = local write "y distance currently being travelled"(0) -> ()
                    n294 = Select(t=T2."nothing", s=w962, f=T2."j") -> (s? t:f=w958:T2)
                    n295 = local write "part"(w958) -> ()
                    "Step 2J" <- TRUE
                  }
                  frame "nothing" {
                    n296 = local write "y distance currently being travelled"(0) -> ()
                    n297 = local write "x distance currently being travelled"(0) -> ()
                  }
                }
              }
              frame True {
                n298 = case shown="\"radius_travel\"" "part circle" {
                  frame "a" {
                    n299 = for {
                      N: 1 -> [_]
                      n300 = local read "Pulses M1"() -> (w976:dbl)
                      n301 = local read "Pulses M2"() -> (w975:dbl)
                      n302 = Equal To 0?(x=w976) -> (x = 0?=w978:bool)
                      n303 = Equal To 0?(x=w975) -> (x = 0?=w979:bool)
                      n304 = And(x=w978, y=w979) -> (x .and. y?=w977:bool)
                      "circle reset" <- w977
                      n305 = Select(t=T1."going right", s=w977, f=T1."a") -> (s? t:f=w973:T1)
                      n306 = local write "Has encoders been reset?"(enum16{"don't reset", "reset"}."reset") -> ()
                      n307 = local write "part circle"(w973) -> ()
                    }
                    n308 = local write "x distance currently being travelled"(0) -> ()
                    n309 = local write "y distance currently being travelled"(0) -> ()
                  }
                  frame "going down" {
                    n310 = local read "calc distance y"() -> (w988:dbl)
                    n311 = Greater?(x=w988, y=19000) -> (0:w986:bool)
                    n312 = local write "Has encoders been reset?"(enum16{"don't reset", "reset"}."don't reset") -> ()
                    n313 = Select(t=T1."going right", s=w986, f=T1."going down") -> (s? t:f=w983:T1)
                    n314 = local write "y distance currently being travelled"(-2) -> ()
                    n315 = local write "x distance currently being travelled"(0) -> ()
                    n316 = local write "part circle"(w983) -> ()
                    "down" <- TRUE
                  }
                  frame "going right" {
                    n317 = for {
                      N: 1 -> [_]
                      n318 = local read "Pulses M1"() -> (w999:dbl)
                      n319 = local read "Pulses M2"() -> (w998:dbl)
                      n320 = Equal To 0?(x=w999) -> (x = 0?=w1001:bool)
                      n321 = Equal To 0?(x=w998) -> (x = 0?=w1002:bool)
                      n322 = And(x=w1001, y=w1002) -> (x .and. y?=w1000:bool)
                      n323 = Select(t=T1."radius_travel", s=w1000, f=T1."going right") -> (s? t:f=w996:T1)
                      n324 = local write "Has encoders been reset?"(enum16{"don't reset", "reset"}."reset") -> ()
                      n325 = local write "part circle"(w996) -> ()
                    }
                    n326 = local write "x distance currently being travelled"(0) -> ()
                    n327 = local write "y distance currently being travelled"(0) -> ()
                    "right" <- TRUE
                  }
                  frame "radius_travel" {
                    n328 = local read "calc distanc x"() -> (w1005:dbl)
                    n329 = local write "x distance currently being travelled"(-4) -> ()
                    n330 = Greater?(x=w1005, y=39000) -> (0:w1009:bool)
                    n331 = local write "Has encoders been reset?"(enum16{"don't reset", "reset"}."don't reset") -> ()
                    n332 = Select(t=T1."going right", s=w1009, f=T1."going down") -> (s? t:f=w1004:T1)
                    n333 = local write "part circle"(w1004) -> ()
                    "down 2" <- TRUE
                  }
                  frame "reset_before_circle" {
                    n334 = local write "x distance currently being travelled"(0) -> ()
                    n335 = local write "y distance currently being travelled"(0) -> ()
                  }
                  frame "circle" {
                    n336 = local write "x distance currently being travelled"(0) -> ()
                    n337 = local write "y distance currently being travelled"(0) -> ()
                  }
                  frame "nothing" {
                    n338 = local write "x distance currently being travelled"(0) -> ()
                    n339 = local write "y distance currently being travelled"(0) -> ()
                  }
                }
              }
            }
            "Numeric" <- 2
          }
        }
      }
    }
    "In drawing mode" <- w166
    n340 = And(x=w77, y=w70) -> (x .and. y?=w148:bool)
    n341 = Or(x=w203, y=w148) -> (x .or. y?=w202:bool)
    n342 = Or(x=w202, y="Motor stop") -> (x .or. y?=w204:bool)
    n343 = Or(x=w204, y="stop") -> (x .or. y?=w224:bool)
    n344 = Select(t=0.0, s=w224, f=w61) -> (s? t:f=w221:dbl)
    n345 = call-poly <vilib>:"DAQmx Write.vi"("task/channels in"=w230, "data"=w221, "error in"=w227) -> ("task out"=w231:refnum<k21>, "error out"=w232:errorcluster)  [unwired: 10 in, 1 out]
    n346 = Select(t=0.0 ("s? t:f"), s=w224, f=w62) -> (s? t:f=w222:dbl)
    n347 = call-poly <vilib>:"DAQmx Write.vi"("task/channels in"=w236, "data"=w222, "error in"=w226) -> ("task out"=w235:refnum<k21>, "error out"=w234:errorcluster)  [unwired: 10 in, 1 out]
    n348 = call <vilib>:"DAQmx Wait Until Done.vi"("task/channels in"=w235, "error in"=w234) -> ("error out"=w233:errorcluster)  [unwired: 12 in, 1 out]
    n349 = call <vilib>:"DAQmx Wait Until Done.vi"("task/channels in"=w231, "error in"=w232) -> ("error out"=w229:errorcluster)  [unwired: 12 in, 1 out]
    n350 = case shown="True" w136 {
      tunnel: w137 -> [w289 w290]
      frame False {
        n351 = call-poly <vilib>:"DAQmx Read.vi"("task/channels in"=w289) -> ("data"=w288:dbl)  [unwired: 12 in, 2 out]
        n352 = local write "Pulses M2"(w288) -> ()
      }
      frame True {
        n353 = local read "Has encoders been reset?"() -> (w291:enum16{"don't reset", "reset"})
        n354 = case shown="\"reset\"" w291 {
          tunnel: w290 -> [w293 w296]
          frame "don't reset", Default {
            n355 = call-poly <vilib>:"DAQmx Read.vi"("task/channels in"=w293) -> ("data"=→"Pulses M2":dbl)  [unwired: 12 in, 2 out]
          }
          frame "reset" {
            n356 = call <vilib>:"DAQmx Stop Task.vi"("task/channels in"=w296) -> ("task out"=w295:refnum<k21>)  [unwired: 13 in, 1 out]
            n357 = call <vilib>:"DAQmx Start Task.vi"("task/channels in"=w295) -> ("task out"=w297:refnum<k21>)  [unwired: 13 in, 1 out]
            n358 = call-poly <vilib>:"DAQmx Read.vi"("task/channels in"=w297) -> ("data"=w294:dbl)  [unwired: 12 in, 2 out]
            n359 = local write "Pulses M2"(w294) -> ()
          }
        }
      }
    }
    n360 = call "Number To Enum.vim"("number"=w162, "enum type"=enum16{"corner", "1st switch", "reverse"}."corner") -> ("number as enum"=→"Shape drawing steps":enum16{"corner", "1st switch", "reverse"})
    n361 = case shown="True" w136 {
      tunnel: w141 -> [w300 w305]
      tunnel: w140 -> [w301 w304]
      tunnel: [w298 w303] -> w139
      frame False {
        n362 = call-poly <vilib>:"DAQmx Read.vi"("task/channels in"=w300, "error in"=w301) -> ("data"=w299:dbl, "error out"=w298:errorcluster)  [unwired: 11 in, 1 out]
        n363 = local write "Pulses M1"(w299) -> ()
      }
      frame True {
        n364 = case shown="\"reset\"" "Has encoders been reset?" {
          tunnel: w305 -> [w309 w316]
          tunnel: w304 -> [w308 w315]
          tunnel: [w306 w317] -> w303
          frame "don't reset", Default {
            n365 = call-poly <vilib>:"DAQmx Read.vi"("task/channels in"=w309, "error in"=w308) -> ("data"=→"Pulses M1":dbl, "error out"=w306:errorcluster)  [unwired: 11 in, 1 out]
          }
          frame "reset" {
            n366 = call <vilib>:"DAQmx Stop Task.vi"("task/channels in"=w316, "error in"=w315) -> ("task out"=w314:refnum<k21>, "error out"=w313:errorcluster)  [unwired: 12 in]
            n367 = call <vilib>:"DAQmx Start Task.vi"("task/channels in"=w314, "error in"=w313) -> ("task out"=w312:refnum<k21>, "error out"=w311:errorcluster)  [unwired: 12 in]
            n368 = call-poly <vilib>:"DAQmx Read.vi"("task/channels in"=w312, "error in"=w311) -> ("data"=w310:dbl, "error out"=w317:errorcluster)  [unwired: 11 in, 1 out]
            n369 = local write "Pulses M1"(w310) -> ()
          }
        }
      }
    }
  }
  n370 = invoke on="motor 1" class="Slide (strict)" method="Reinit To Default"() -> ()  [unwired: 3 in, 3 out]
  n371 = call <vilib>:"Simple Error Handler.vi"("error source (\" \")"="you messed up" ("error source (\" \")"), "error in (no error)"=w48) -> ()  [unwired: 3 in, 5 out]
  n372 = call <vilib>:"Simple Error Handler.vi"("error source (\" \")"="you messed up" ("error source (\" \")"), "error in (no error)"=w45) -> ()  [unwired: 3 in, 5 out]
  n373 = call <vilib>:"DAQmx Clear Task.vi"("task in"=w27, "error in"=w25) -> ()  [unwired: 13 in, 1 out]
  n374 = call <vilib>:"DAQmx Clear Task.vi"("task in"=w17, "error in"=w14) -> ()  [unwired: 13 in, 1 out]
  n375 = call <vilib>:"DAQmx Clear Task.vi"("task in"=w18, "error in"=w15) -> ("error out"=w12:errorcluster)  [unwired: 13 in]
  n376 = call <vilib>:"DAQmx Clear Task.vi"("task in"=w16, "error in"=w13) -> ()  [unwired: 13 in, 1 out]
  n377 = call <vilib>:"Simple Error Handler.vi"("error in (no error)"=w12) -> ()  [unwired: 4 in, 5 out]
  n378 = call <vilib>:"Simple Error Handler.vi"("error source (\" \")"="you messed up" ("error source (\" \")"), "error in (no error)"=w10) -> ()  [unwired: 3 in, 5 out]
